vi "Read driver_param.vi"(8 "error in (no error)":errorcluster, 11 "SMSD in":refnum<class "SMSD.lvclass">) -> (0 "error out":errorcluster, 2 "Driver_param":T1={"min_speed"=0, "max_speed"=15600, "acc"=6400, "dec"=6400} {"dec" min=15 max=59000 step=1; "acc" min=15 max=59000 step=1; "max_speed" min=16 max=15600 step=1; "min_speed" max=950 step=1}, 3 "SMSD out":refnum<class "SMSD.lvclass">)   [LabVIEW 2019, in "SMSD.lvclass"]
uses:
  SMSD.lvclass
  SMSD.lvclass/SMSD.ctl
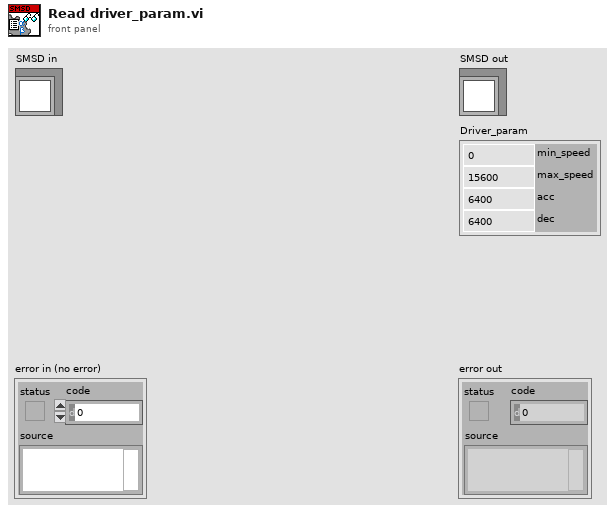
[diagram p1: front panel]
types:
  T1 = cluster{"min_speed":u32, "max_speed":u32, "acc":u32, "dec":u32}
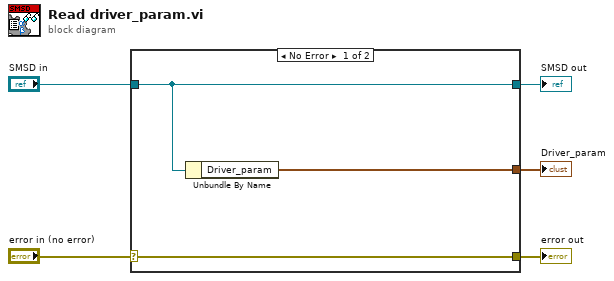
[diagram p0: block diagram]
diagram:
  n1 = case shown="No Error" "error in (no error)" {
    selector: "error in (no error)" -> [w8 w9]
    tunnel: [w8 w9] -> w4
    tunnel: [w7 w10] -> w2
    tunnel: "SMSD in" -> [w7 w10]
    tunnel: [w6 _] -> w1
    frame No Error {
      n2 = Unbundle By Name(w7) -> ("Driver_param"=w6:T1)
    }
    frame Error {
    }
  }
  "error out" <- w4
  "SMSD out" <- w2
  "Driver_param" <- w1
